vi "DG535.get T0 amplitude.vi"(0 "i ref in":refnum<vi>, 11 "error in (no error)":errorcluster) -> (4 "i ref out":refnum<vi>, 8 "amplitude":dbl=1.0 min=-3.0 max=4.0 format="%.2f", 15 "error out":errorcluster)   [LabVIEW 2014, in "DG535.lvlib"]
uses:
  DG535.lvlib
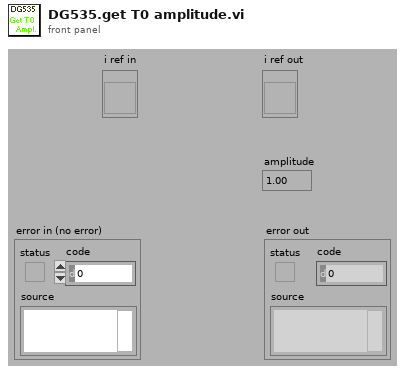
[diagram p1: front panel]
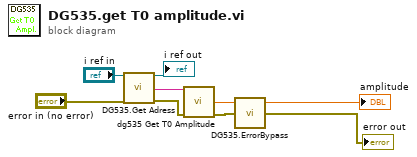
[diagram p0: block diagram]
diagram:
  n1 = call "DG535.Get Adress.vi"("i ref in"="i ref in", "error in (no error)"="error in (no error)") -> ("i ref out"=→"i ref out":refnum<vi>, "address"=w5:string, "error out"=w4:errorcluster)  [unwired: 10 in, 1 out]
  n2 = call "dg535 Get T0 Amplitude.vi"("address string"=w5, "error in"=w4) -> ("amplitude"=→"amplitude":dbl, "error out"=w2:errorcluster)  [unwired: 12 in]
  n3 = call "DG535.ErrorBypass.vi"("error in (no error)"=w2) -> ("error out"=→"error out":errorcluster)  [unwired: 14 in]
